vi "10-Tap 8-bit Camera with DRAM (Host).vi"() -> ()   [LabVIEW 2013]
doc: "This is the host VI for the 10-Tap 8-Bit Camera with DRAM example. This example demonstrates how to acquire images from a 10-tap, 8-bit, extended configuration, Camera Link camera and display the images on the host. This example supports area scan and line scan cameras for both continuous and finite acquisitions.\n\nThis example also demonstrates the use of DRAM as a frame buffer for very high speed acquisitions. Data packing and flow-control are also employed to maximize use of the available DRAM and FIFOs in terms of both memory space and performance.\n\nAdditionally, the example demonstrates the serial server, which allows third-party camera configuration utilities to communicate with the camera using the Camera Link serial interface while this VI is running."
uses:
  <vilib>/rvi/interface/nirviOpenFPGA/nirviOpenFPGA.xnode
  <vilib>/rvi/interface/nirviMethod/nirviMethod.xnode
  <vilib>/rvi/interface/nirviCloseFPGA/nirviCloseFPGA.xnode
  <vilib>/rvi/interface/nirviReadWriteControl/nirviReadWriteControl.xnode
  <vilib>/rvi/interface/Simulation/niFpgaSimulationCallBeginRW.vi
  <vilib>/rvi/errors/niLvFpgaAdjustHostInterfaceError.vi
  <vilib>/rvi/errors/niLvFpgaMergeErrorWithErrorCode.vi
  <vilib>/FPGAPlugInAG/Dynamic/niLvFpga_Reset_Dynamic.vi
  <vilib>/FPGAPlugInAG/Dynamic/niLvFpga_Run_Dynamic.vi
  <vilib>/FPGAPlugInAG/Dynamic/niLvFpga_ConfigureFifo_Dynamic.vi
  <vilib>/FPGAPlugInAG/Dynamic/niLvFpga_StartFifo_Dynamic.vi
  <vilib>/FPGAPlugInAG/Dynamic/niLvFpga_ReadFifo_Dynamic.vi
  <vilib>/FPGAPlugInAG/Dynamic/niLvFpga_WriteFifo_Dynamic.vi
  <vilib>/FPGAPlugInAG/Dynamic/niLvFpga_StopFifo_Dynamic.vi
  FPGA Bitfiles/10-Tap8-bitwithout_DRAM.lvbitx
  10-Tap 8-bit Camera with DRAM v2 (FPGA).vi
  <vilib>/FPGAPlugInAG/Dynamic/niLvFpga_Close_Dynamic.vi
  <vilib>/userdefined/High Color/nirio_resource_hc.ctl
panel:
  out "Data 2":u64[](array[numeric])
  out "output array 2":u8[][](array[numeric])
  out "Elements Remaining":u32
  out "Data":u64[](array[numeric])
  out "10Pixel values":T1(array[cluster])
  out "output array":u8[](array[numeric])
  out "Y Resolution":i32
  out "X Resolution":i32
  in  "Test Image Path":path=path "C:/Users/achiu/Desktop/testflyimage1.jpg"
  in  "Sim?":bool=TRUE
  in  "DMA Buffer Size\n(In Images)":u32=64 caption="DMA Buffer Size"
  in  "Signal Mapping":T2(ring)=enum."Basler 10-tap"
  out "Acq In Progress":bool
  in  "Line Scan":bool
  in  "Frames To Acquire":u32=1 caption="Frames To Acquire\n(0 = infinite)"
  in  "Cancel":bool
  out "Acq'd Frame Width":u32
  in  "Stopped":bool
  in  "RIO Device":T3="RIO1"
  out "DMA Write Timeout":bool
  in  "Start Serial Server":bool
  out "Frames Acq'd":u32
  out "Acq'd Frame Height":u32
  out "Image":T4(plugin-control)
  in  "Acquire":bool
  in  "Stop":bool
  in  "Image Height":u32=100 max=65535
  in  "Image Width":u32=120 max=65535 step=40
  out "Initialized":bool
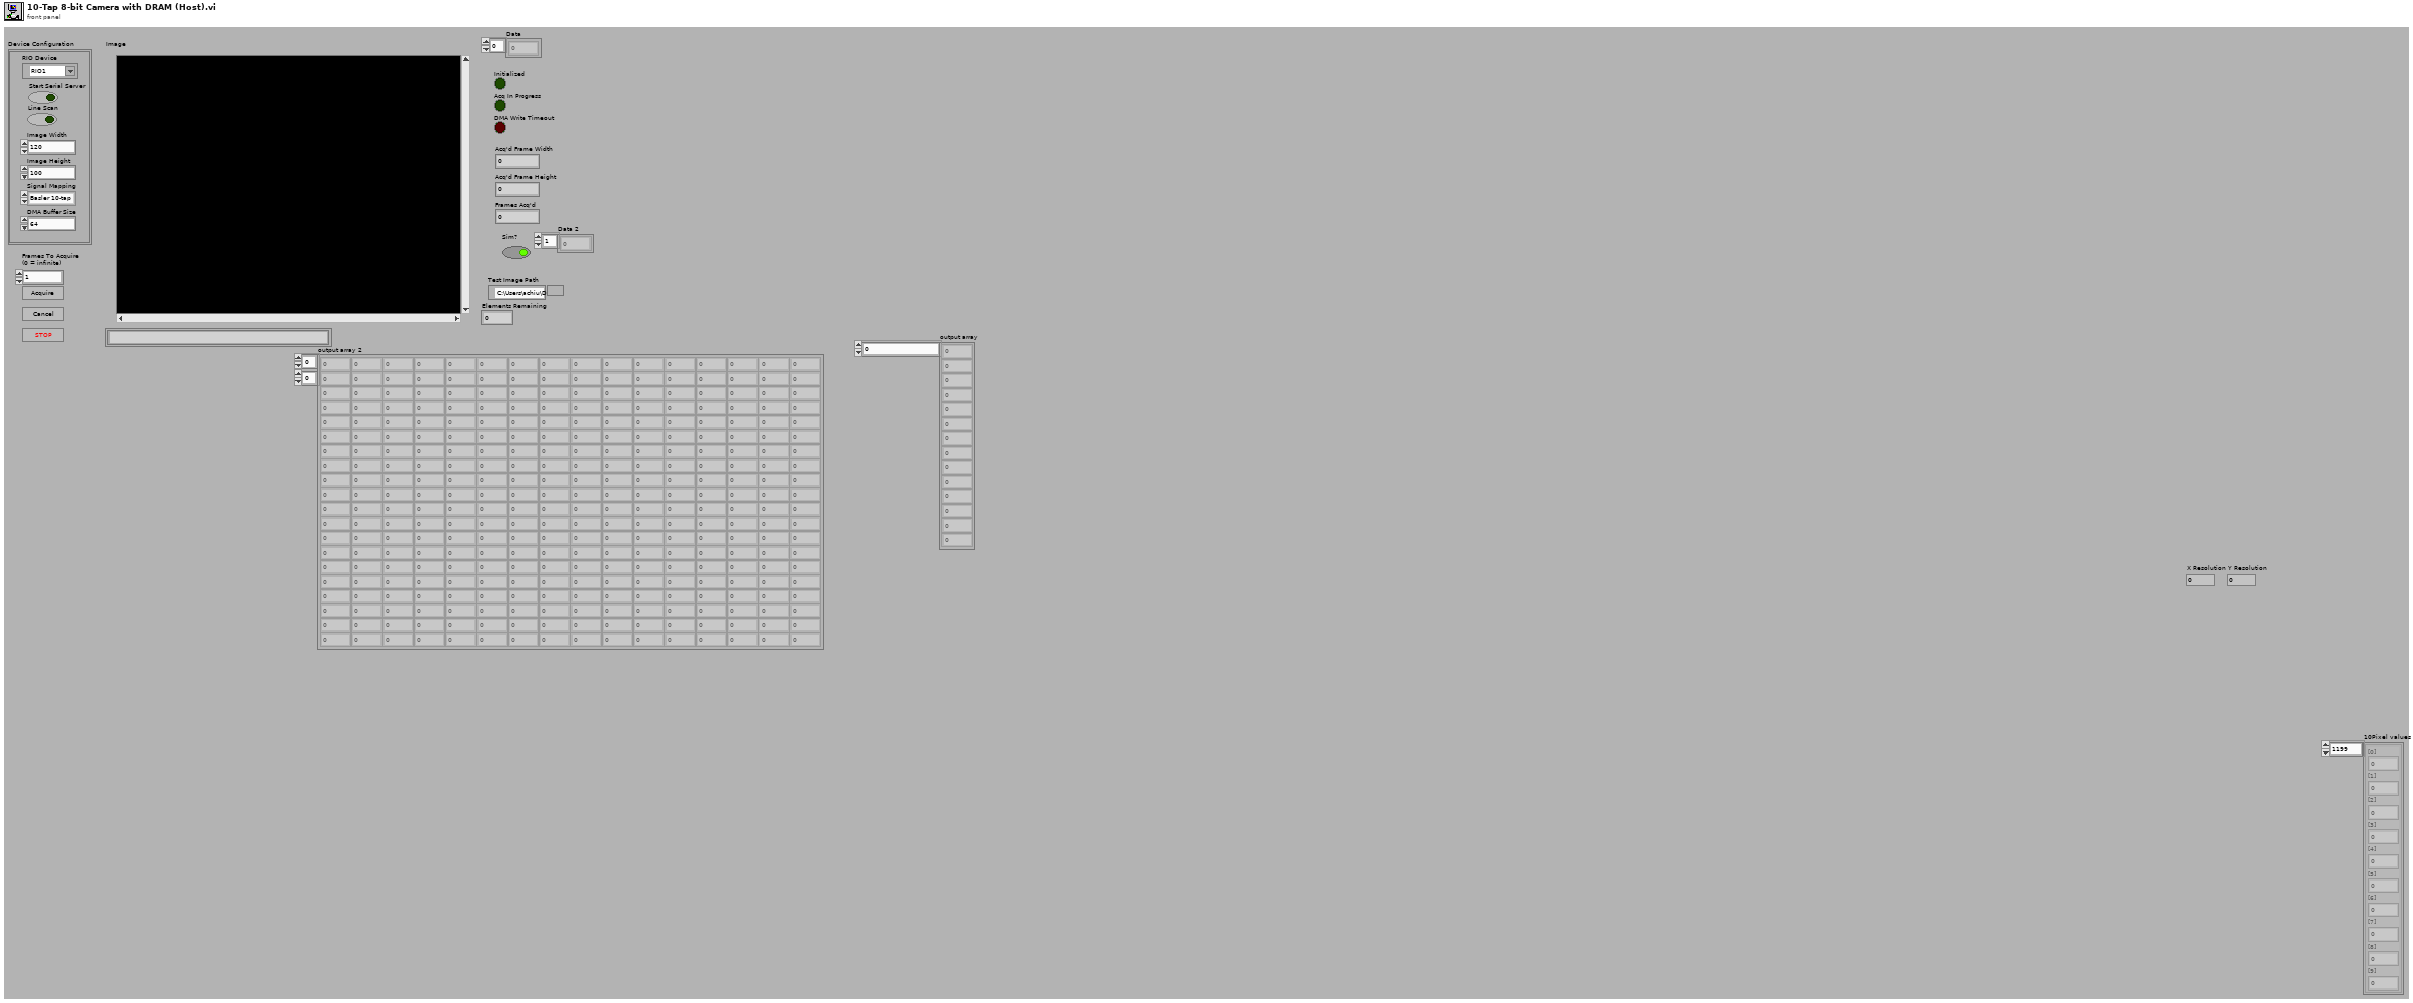
[diagram p1: front panel]
types:
  T1 = cluster{"[0]":u8, "[1]":u8, "[2]":u8, "[3]":u8, "[4]":u8, "[5]":u8, "[6]":u8, "[7]":u8, "[8]":u8, "[9]":u8}[]
  T2 = enum8{"Standard", "Basler 10-tap", "Vosskühler 10-tap"}
  T3 = typedef "nirio_resource_hc.ctl" = tag
  T4 = typedef "IMAQ Image.ctl" = refnum<image>
  T5 = typedef "Image Type" = u32
  T6 = cluster{"[0]":u8, "[1]":u8, "[2]":u8, "[3]":u8, "[4]":u8, "[5]":u8, "[6]":u8, "[7]":u8, "[8]":u8, "[9]":u8}
  T7 = enum16{"big-endian, network order", "native, host order", "little-endian"}
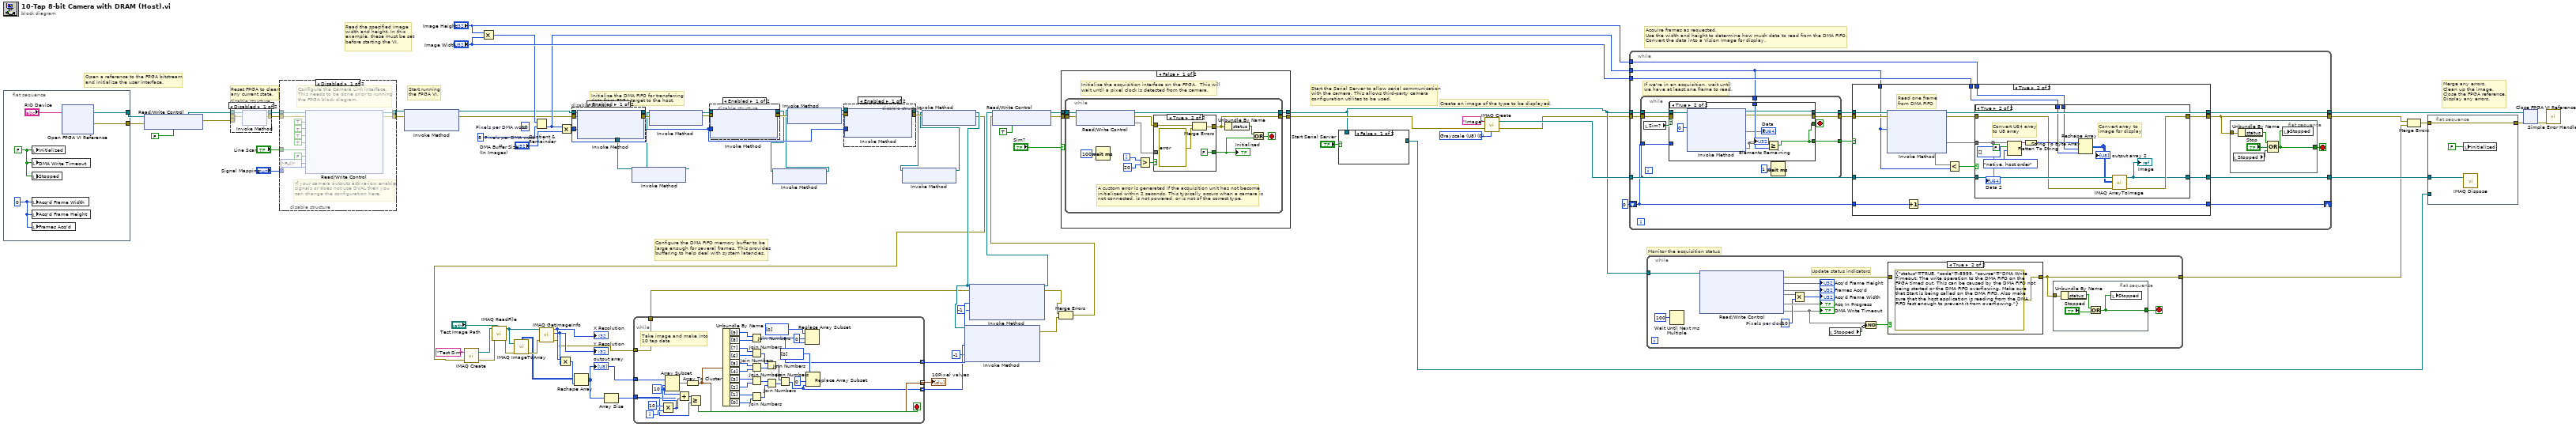
[diagram p0: block diagram]
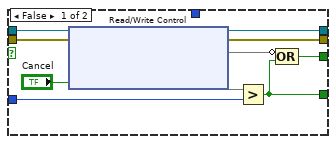
[diagram p3: hidden frame]
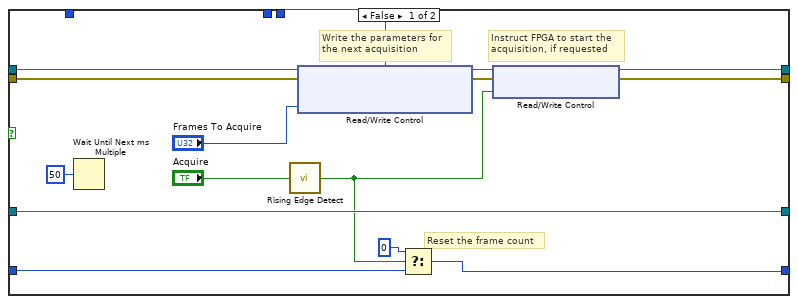
[diagram p4: hidden frame]
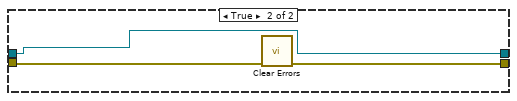
[diagram p12: hidden frame]
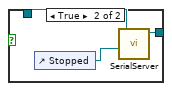
[diagram p13: hidden frame]
diagram:
  w19 = u32 8  # Pixels per DMA word
  (unwired) u32 10  # Pixels per DMA word
  w76 = T5 0 items=["Grayscale (U8)", "Grayscale (I16)", "Grayscale (SGL)", "Complex (CSG)", "RGB (U32)", "HSL (U32)", "RGB (U64)", "Grayscale (U16)"] ("Image Type")
  # "Acquire frames as requested.\nUse the width and height to determine how much data to read from the DMA FIFO.\nConvert the data into a Vision Image for display."
  # "Monitor the acquisition status"
  # "Initialize the DMA FIFO for transferring\ndata from FPGA target to the host."
  # "Configure the DMA FIFO memory buffer to be\nlarge enough for several frames. This provides\nbuffering to help deal with system latencies."
  # "Start running\nthe FPGA VI."
  # "Reset FPGA to clear\nany current state."
  # "Read the specified image\nwidth and height. In this\nexample, these must be set\nbefore starting the VI."
  # "Merge any errors.\nClean up the image.\nClose the FPGA reference.\nDisplay any errors."
  # "Start the Serial Server to allow serial communication\nwith the camera. This allows third-party camera\nconfiguration utilites to be used."
  # "Create an image of the type to be displayed."
  # "Open a reference to the FPGA bitstream\nand initialize the user interface."
  n1 = flat-sequence {
    tunnel: [w81] -> w6
    tunnel: [w80] -> w7
    frame #0 {
      w84 = u32 0 ("Num Lines Acq'd")
      w83 = FALSE ("stop")
      n2 = local write "Initialized"(w83) -> ()
      n3 = local write "DMA Write Timeout"(w83) -> ()
      n4 = local write "Stopped"(w83) -> ()
      n5 = local write "Acq'd Frame Width"(w84) -> ()
      n6 = local write "Acq'd Frame Height"(w84) -> ()
      n7 = local write "Frames Acq'd"(w84) -> ()
      n8 = xnode "Open FPGA VI Reference"("resource name"="RIO Device") -> ("FPGA VI Reference Out"=w81:refnum<k20>, "error out"=w80:errorcluster)  [unwired: 1 in]
    }
  }
  n9 = xnode "Read/Write Control"("FPGA VI Reference In"=w6, "error in"=w7, "Acq Control.Initialize"=FALSE ("Arm Acquisition")) -> ("FPGA VI Reference Out"=w5:refnum<k20>, "error out"=w4:errorcluster)
  n10 = disable-structure shown="Disabled" {
    disable-tunnel: [w85 _] -> _
    disable-tunnel: w5 -> [w88 w89]
    disable-tunnel: [w87 _] -> w64
    disable-tunnel: [w86 w89] -> w63
    disable-tunnel: w4 -> [w85 _]
    frame Disabled {
      n11 = xnode "Invoke Method"("FPGA VI Reference In"=w88, "error in"=w85) -> ("FPGA VI Reference Out"=w86:refnum<k20>, "error out"=w87:errorcluster)
    }
    frame Enabled {
    }
  }
  n12 = disable-structure shown="Disabled" {
    disable-tunnel: [w101 w103] -> w31
    disable-tunnel: w64 -> [w100 w102]
    disable-tunnel: [w99 w102] -> w30
    disable-tunnel: w63 -> [w98 w103]
    disable-tunnel: "Line Scan" -> [w93 _]
    disable-tunnel: "Signal Mapping" -> [w90 _]
    frame Disabled {
      # "If your camera outputs active-low enable\nsignals or does not use DVAL then you \ncan change the configuration here."
      # "Configure the Camera Link interface.\nThis needs to be done prior to running\nthe FPGA block diagram."
      n13 = xnode "Read/Write Control"("FPGA VI Reference In"=w98, "error in"=w100, "CL Config.FVAL Active High"=TRUE ("IO Module Config.CL FVAL Active High"), "CL Config.LVAL Active High"=TRUE ("IO Module Config.CL LVAL Active High"), "CL Config.DVAL Active High"=TRUE ("IO Module Config.CL DVAL Active High"), "CL Config.Spare Active High"=TRUE ("IO Module Config.CL Spare Active High"), "CL Config.Line Scan"=w93, "Acq Control.Ignore DVAL"=FALSE ("CL Config.Line Scan"), "CL Config.Configuration"=enum8{"Base", "Medium", "Full"}."Full", "CL Config.Signal Mapping"=w90) -> ("FPGA VI Reference Out"=w101:refnum<k20>, "error out"=w99:errorcluster)
    }
    frame Enabled {
    }
  }
  n14 = xnode "Invoke Method"("FPGA VI Reference In"=w31, "error in"=w30) -> ("FPGA VI Reference Out"=w29:refnum<k20>, "error out"=w28:errorcluster)  [unwired: 1 in]
  n15 = Multiply(x="Image Height", y="Image Width") -> (x*y=w57:u32)
  n16 = Quotient & Remainder(x=w57, y=w19) -> (floor(x/y)=w56:u32)  [unwired: 1 out]
  n17 = Multiply(x=w56, y="DMA Buffer Size\n(In Images)") -> (x*y=w55:u32)
  n18 = disable-structure shown="Enabled" {
    disable-tunnel: w29 -> [w108 w110]
    disable-tunnel: w28 -> [w107 w109]
    disable-tunnel: w55 -> [w106 _]
    disable-tunnel: [w104 w110] -> _
    disable-tunnel: [w105 w109] -> w39
    disable-tunnel: [w104 _] -> w25
    frame Enabled {
      n19 = xnode "Invoke Method"("FPGA VI Reference In"=w108, "error in"=w107, "Requested Depth"=w106) -> ("FPGA VI Reference Out"=w104:refnum<k20>, "error out"=w105:errorcluster)  [unwired: 1 out]
    }
    frame Disabled {
    }
  }
  n20 = xnode "Invoke Method"("FPGA VI Reference In"=w25) -> ("FPGA VI Reference Out"=w24:refnum<k20>)  [unwired: 1 in, 1 out]
  n21 = xnode "Invoke Method"("FPGA VI Reference In"=w24, "error in"=w39) -> ("FPGA VI Reference Out"=w37:refnum<k20>, "error out"=w35:errorcluster)
  n22 = disable-structure shown="Enabled" {
    disable-tunnel: w55 -> [w115 _]
    disable-tunnel: w37 -> [w114 w117]
    disable-tunnel: [w113 w117] -> w23
    disable-tunnel: [w112 w116] -> w36
    disable-tunnel: w35 -> [w111 w116]
    frame Enabled {
      n23 = xnode "Invoke Method"("FPGA VI Reference In"=w114, "error in"=w111, "Requested Depth"=w115) -> ("FPGA VI Reference Out"=w113:refnum<k20>, "error out"=w112:errorcluster)  [unwired: 1 out]
    }
    frame Disabled {
    }
  }
  n24 = xnode "Invoke Method"("FPGA VI Reference In"=w23) -> ("FPGA VI Reference Out"=w22:refnum<k20>)  [unwired: 1 in, 1 out]
  n25 = xnode "Invoke Method"("FPGA VI Reference In"=w22, "error in"=w36) -> ("FPGA VI Reference Out"=w34:refnum<k20>, "error out"=w33:errorcluster)
  n26 = disable-structure shown="Enabled" {
    disable-tunnel: w55 -> [w122 _]
    disable-tunnel: w34 -> [w121 w124]
    disable-tunnel: w33 -> [w120 w123]
    disable-tunnel: [w119 w124] -> w21
    disable-tunnel: [w118 w123] -> w32
    frame Enabled {
      n27 = xnode "Invoke Method"("FPGA VI Reference In"=w121, "error in"=w120, "Requested Depth"=w122) -> ("FPGA VI Reference Out"=w119:refnum<k20>, "error out"=w118:errorcluster)  [unwired: 1 out]
    }
    frame Disabled {
    }
  }
  n28 = xnode "Invoke Method"("FPGA VI Reference In"=w21) -> ("FPGA VI Reference Out"=w20:refnum<k20>)  [unwired: 1 in, 1 out]
  n29 = xnode "Invoke Method"("FPGA VI Reference In"=w20, "error in"=w32) -> ("FPGA VI Reference Out"=w14:refnum<k20>, "error out"=w13:errorcluster)
  n30 = call "IMAQ Create"("Image Name"="Test Sim", "error in (no error)"=w13) -> ("New Image"=w51:T4, "error out"=w50:errorcluster)  [unwired: 3 in]
  n31 = call "IMAQ ReadFile"("File Path"="Test Image Path", "error in (no error)"=w50, "Image"=w51) -> ("error out"=w45:errorcluster, "Image Out"=w49:T4)  [unwired: 4 in, 3 out]
  n32 = call "IMAQ ImageToArray"("error in (no error)"=w45, "Image"=w49) -> ("error out"=w44:errorcluster, "Image Pixels (U8)"=w1:u8[][])  [unwired: 2 in, 3 out]
  n33 = call "IMAQ GetImageInfo"("error in (no error)"=w44, "Image"=w49) -> ("error out"=w40:errorcluster, "Y Resolution"=w42:i32, "X Resolution"=w43:i32)  [unwired: 2 in, 5 out]
  "X Resolution" <- w43
  "Y Resolution" <- w42
  n34 = Multiply(x=w43, y=w42) -> (x*y=w41:i32)
  n35 = Reshape Array(w1, w41) -> (w47:u8[])
  "output array" <- w47
  n36 = Array Size(array=w47) -> (size(s)=w48:i32)
  n37 = while {
    tunnel: w48 -> [w150]
    tunnel: w47 -> [w155]
    tunnel: [w132] -> w46 mode=indexing
    tunnel: w40 -> [w125]
    tunnel: [w127] -> w27 mode=indexing
    tunnel: [w126] -> w26 mode=indexing
    tunnel: [w125] -> w8
    i -> [w157]
    stop <- w149 stop-if-true
    w152 = 10 ("length")
    # "Take image and make into\n10 tap data"
    n38 = Multiply(x=10, y=w157) -> (x*y=w153:i32)
    n39 = Array Subset(array=w155, index=w153, length=w152) -> (w154:u8[])
    n40 = Add(x=w152, y=w153) -> (x+y=w151:i32)
    n41 = Array To Cluster(array=w154) -> (cluster=w132:T6)
    n42 = Greater Or Equal?(x=w151, y=w150) -> (x >= y?=w149:bool)
    n43 = Unbundle By Name(w132) -> ("[9]"=w148:u8, "[8]"=w147:u8, "[7]"=w146:u8, "[6]"=w145:u8, "[5]"=w144:u8, "[4]"=w143:u8, "[3]"=w142:u8, "[2]"=w141:u8, "[1]"=w140:u8, "[0]"=w139:u8)
    n44 = Join Numbers(hi=w148, lo=w147) -> ((hi.lo)=w127:u16)
    n45 = Join Numbers(hi=w146, lo=w145) -> ((hi.lo)=w137:u16)
    n46 = Join Numbers(hi=w144, lo=w143) -> ((hi.lo)=w136:u16)
    n47 = Join Numbers(hi=w142, lo=w141) -> ((hi.lo)=w135:u16)
    n48 = Join Numbers(hi=w140, lo=w139) -> ((hi.lo)=w138:u16)
    n49 = Join Numbers(hi=w137, lo=w136) -> ((hi.lo)=w134:u32)
    n50 = Join Numbers(hi=w135, lo=w138) -> ((hi.lo)=w133:u32)
    n51 = Join Numbers(hi=w134, lo=w133) -> ((hi.lo)=w126:u64)
    n52 = Replace Array Subset(array=u16[] [0] ("Data"), new element=w127, index=0) -> ()  [unwired: 1 out]
    n53 = Replace Array Subset(array=u64[] [0] ("Data"), new element=w126, index=0) -> ()  [unwired: 1 out]
  }
  "10Pixel values" <- w46
  n54 = xnode "Invoke Method"("FPGA VI Reference In"=w14, "Data"=w26, "Timeout (ms)"=-1) -> ("error out"=w11:errorcluster)  [unwired: 1 in, 2 out]
  n55 = xnode "Invoke Method"("FPGA VI Reference In"=w14, "error in"=w8, "Data"=w27, "Timeout (ms)"=-1) -> ("FPGA VI Reference Out"=w9:refnum<k20>, "error out"=w12:errorcluster)  [unwired: 1 out]
  n56 = Merge Errors(w12, w11) -> (w10:errorcluster)
  n57 = xnode "Read/Write Control"("FPGA VI Reference In"=w9, "error in"=w10, "Acq Control.Initialize"=TRUE ("Arm Acquisition")) -> ("FPGA VI Reference Out"=w79:refnum<k20>, "error out"=w78:errorcluster)
  n58 = case shown="False" "Sim?" {
    tunnel: w79 -> [w161 w181]
    tunnel: w78 -> [w160 w182]
    tunnel: [w159 w181] -> w18
    tunnel: [w158 w183] -> w61
    frame False {
      # "Initialize the acquisition interface on the FPGA.  This will\nwait until a pixel clock is detected from the camera."
      n59 = while {
        tunnel: w161 -> [w169]
        tunnel: w160 -> [w168]
        tunnel: [w167] -> w159
        tunnel: [w171] -> w158
        i -> [w163]
        stop <- w174 stop-if-true
        # "A custom error is generated if the acquisition unit has not become\ninitialized within 2 seconds. This typically occurs when a camera is\nnot connected, is not powered, or is not of the correct type."
        n60 = xnode "Read/Write Control"("FPGA VI Reference In"=w169, "error in"=w168) -> ("FPGA VI Reference Out"=w167:refnum<k20>, "error out"=w166:errorcluster, "Acq Status.Initialized"=w165)
        n61 = Wait (ms)(milliseconds to wait=u32 100) -> ()  [unwired: 1 out]
        n62 = Greater?(x=w163, y=20) -> (0:w164:bool)
        n63 = case shown="True" w164 {
          tunnel: [w176 FALSE] -> w170
          tunnel: w165 -> [w176 _]
          tunnel: w166 -> [w175 w178]
          tunnel: [w175 w180] -> w171
          frame False {
          }
          frame True {
            n64 = Merge Errors(w178, errorcluster {"status"=TRUE, "code"=-8999, "source"="Acquisition Initialization: This error typically occurs when a camera is not properly connected, is not powered, or is not of the correct type."} ("error in")) -> (w180:errorcluster)
          }
        }
        "Initialized" <- w170
        n65 = Unbundle By Name(w171) -> ("status"=w173:bool)
        n66 = Or(x=w173, y=w170) -> (x .or. y?=w174:bool)
      }
    }
    frame True {
      n67 = call <vilib>:"Clear Errors.vi"("error in (no error)"=w182) -> ("error out"=w183:errorcluster)  [unwired: 6 in]
    }
  }
  n68 = case shown="False" "Start Serial Server" {
    tunnel: [_ w184] -> w68
    tunnel: w18 -> [_ w185]
    frame False {
    }
    frame True {
      n69 = control-ref of="Stopped"() -> (w186:refnum<vi>)
      n70 = call "SerialServer.vi"("Stop Refnum"=w186, "FPGA VI Reference In"=w185) -> ("FPGA VI Reference Out"=w184:refnum<k20>)  [unwired: 5 in]
    }
  }
  n71 = call "IMAQ Create"("Image Name"="Image", "Image Type"=w76, "error in (no error)"=w61) -> ("New Image"=w59:T4, "error out"=w15:errorcluster)  [unwired: 2 in]
  n72 = while {
    tunnel: w18 -> [w194]
    tunnel: w15 -> [w193]
    tunnel: w56 -> [w187]
    tunnel: "Image Height" -> [w201]
    tunnel: "Image Width" -> [w200]
    tunnel: w59 -> [w199]
    tunnel: [w197] -> w66
    tunnel: [w198] -> w75
    tunnel: [w195] -> w70
    shift-right: [w189] -> _
    shift-left: u32 0 -> [w188]
    stop <- w196 stop-if-true
    # "If we're in an acquisition, wait until\nwe have at least one frame to read."
    n73 = while {
      tunnel: w194 -> [w208]
      tunnel: w193 -> [w207]
      tunnel: [w205] -> w192
      tunnel: [w206] -> w191
      tunnel: w188 -> [w211]
      tunnel: [w209] -> w190
      tunnel: w187 -> [w203]
      stop <- w210 stop-if-true
      n74 = local read "Sim?"() -> (w204:bool)
      n75 = case shown="True" w204 {
        tunnel: w211 -> [w221 _]
        tunnel: [w220 w222] -> w210
        tunnel: [w219 w222] -> w209
        tunnel: w208 -> [w218 w229]
        tunnel: w207 -> [w217 _]
        tunnel: [w216 w225] -> w206
        tunnel: [w215 w224] -> w205
        tunnel: w203 -> [_ w226]
        frame False {
          n76 = xnode "Read/Write Control"("FPGA VI Reference In"=w218, "error in"=w217, "Acq Control.Cancel Acq"="Cancel") -> ("FPGA VI Reference Out"=w216:refnum<k20>, "error out"=w215:errorcluster, "Acq Status.Acq In Progress"=w214, "Acq Status.Frames Acq'd"=w213)
          n77 = Greater?(x=w213, y=w221) -> (0:w219:bool)
          n78 = Compound Arithmetic op=OR(invert w214, w219) -> (w220:bool)
        }
        frame True {
          n79 = xnode "Invoke Method"("FPGA VI Reference In"=w229, "Number of Elements"=u32 0) -> ("FPGA VI Reference Out"=w225:refnum<k20>, "error out"=w224:errorcluster, "Data"=→"Data":void[], "Elements Remaining"=w227)  [unwired: 2 in]
          "Elements Remaining" <- w227
          n80 = Greater Or Equal?(x=w227, y=w226) -> (x >= y?=w222:bool)
        }
      }
      n81 = Wait (ms)(milliseconds to wait=u32 1) -> ()  [unwired: 1 out]
    }
    n82 = case shown="True" w190 {
      tunnel: w191 -> [w245 w257]
      tunnel: w192 -> [w244 w256]
      tunnel: w187 -> [_ w250]
      tunnel: w201 -> [w238 w264]
      tunnel: w200 -> [_ w263]
      tunnel: w199 -> [w249 w262]
      tunnel: [w240 w260] -> w197
      tunnel: [w243 w259] -> w198
      tunnel: [w249 w258] -> w195
      tunnel: w188 -> [w246 w255]
      tunnel: [w248 w254] -> w189
      frame False {
        # "Reset the frame count"
        # "Instruct FPGA to start the\nacquisition, if requested"
        # "Write the parameters for\nthe next acquisition"
        n83 = Wait Until Next ms Multiple(millisecond multiple=u32 50) -> ()  [unwired: 1 out]
        n84 = call "Rising Edge Detect.vi"("Input"="Acquire") -> ("Pulse"=w235:bool)  [unwired: 4 in]
        n85 = xnode "Read/Write Control"("FPGA VI Reference In"=w245, "error in"=w244, "Acq Control.Line Scan Height"=w238, "Acq Control.Frames To Acq"="Frames To Acquire") -> ("FPGA VI Reference Out"=w242:refnum<k20>, "error out"=w241:errorcluster)
        n86 = Select(t=u32 0, s=w235, f=w246) -> (s? t:f=w248:u32)
        n87 = xnode "Read/Write Control"("FPGA VI Reference In"=w242, "error in"=w241, "Acq Control.Acquire"=w235) -> ("FPGA VI Reference Out"=w243:refnum<k20>, "error out"=w240:errorcluster)
      }
      frame True {
        # "Read one frame\nfrom DMA FIFO"
        n88 = xnode "Invoke Method"("FPGA VI Reference In"=w257, "error in"=w256, "Number of Elements"=w250) -> ("FPGA VI Reference Out"=w259:refnum<k20>, "error out"=w261:errorcluster, "Data"=w253:void[], "Elements Remaining"=w251)  [unwired: 1 in]
        n89 = Increment(x=w255) -> (x+1=w254:u32)
        n90 = Less?(x=w251, y=w250) -> (x < y?=w252:bool)
        n91 = case shown="True" w252 {
          tunnel: w264 -> [_ w278]
          tunnel: w263 -> [_ w277]
          tunnel: w262 -> [w266 w276]
          tunnel: w261 -> [w265 w275]
          tunnel: [w265 w274] -> w260
          tunnel: [w266 w273] -> w258
          tunnel: w253 -> [_ w270]
          frame False {
            # "Do not display the image if we're falling behind in the acquisition."
          }
          frame True {
            (unwired) u64[] [] ("Data")
            # "Convert U64 array\nto U8 array"
            # "Convert array to\nimage for display"
            n92 = Flatten To String(anything=w270, prepend array or string size? (T)=FALSE, byte order (0:big-endian, network order)=T7."native, host order") -> (data string=w268:string)  [unwired: 1 in, 2 out]
            n93 = String To Byte Array(string=w268) -> (unsigned byte array=w267:u8[])
            n94 = Reshape Array(w267, w278, w277) -> (w272:u8[][])
            "output array 2" <- w272
            n95 = call "IMAQ ArrayToImage"("error in (no error)"=w275, "Image Pixels (U8)"=w272, "Image"=w276) -> ("error out"=w274:errorcluster, "Image Out"=w273:T4)  [unwired: 7 in]
            "Image" <- w273
            "Data 2" <- w270
          }
        }
      }
    }
    n96 = flat-sequence {
      tunnel: w197 -> [w232]
      tunnel: [w231] -> w196
      frame #0 {
        n97 = local read "Stopped"() -> (w230:bool)
        n98 = Unbundle By Name(w232) -> ("status"=w233:bool)
        n99 = Compound Arithmetic op=OR(w233, "Stop", w230) -> (w231:bool)
        n100 = local write "Stopped"(w231) -> ()
      }
    }
  }
  n101 = while {
    tunnel: w18 -> [w289]
    tunnel: [w292] -> w65
    stop <- w291 stop-if-true
    w282 = u32 10  # Pixels per clock
    # "Update status indicators"
    n102 = Wait Until Next ms Multiple(millisecond multiple=u32 100) -> ()  [unwired: 1 out]
    n103 = xnode "Read/Write Control"("FPGA VI Reference In"=w289) -> ("error out"=w288:errorcluster, "Acq Status.Lines Per Frame"=→"Acq'd Frame Height", "Acq Status.Frames Acq'd"=→"Frames Acq'd", "Acq Status.Clocks Per Line"=w283, "Acq Status.Acq In Progress"=→"Acq In Progress", "Acq Status.DMA Write Timeout"=w280)  [unwired: 1 in, 1 out]
    "DMA Write Timeout" <- w280
    n104 = Multiply(x=w283, y=w282) -> (x*y=→"Acq'd Frame Width":u32)
    n105 = local read "Stopped"() -> (w279:bool)
    n106 = Compound Arithmetic op=AND(w280, invert w279) -> (w281:bool)
    n107 = case shown="True" w281 {
      tunnel: w288 -> [w297 _]
      tunnel: [w297 errorcluster {"status"=TRUE, "code"=-8999, "source"="DMA Write Timeout: The write operation to the DMA FIFO on the FPGA timed out. This can be caused by the DMA FIFO not being started or the DMA FIFO overflowing. Make sure that Start is being called on the DMA FIFO. Also make sure that the host application is reading from the DMA FIFO fast enough to prevent it from overflowing."} ("error out")] -> w292
      frame False {
      }
      frame True {
      }
    }
    n108 = flat-sequence {
      tunnel: w292 -> [w296]
      tunnel: [w294] -> w291
      frame #0 {
        n109 = Unbundle By Name(w296) -> ("status"=w295:bool)
        n110 = Or(x=w295, y="Stopped") -> (x .or. y?=w294:bool)
        n111 = local write "Stopped"(w294) -> ()
      }
    }
  }
  n112 = Merge Errors(w66, w65) -> (w67:errorcluster)
  n113 = flat-sequence {
    tunnel: w67 -> [w300]
    tunnel: [w300] -> w72
    tunnel: w70 -> [w301]
    tunnel: w68 -> [_]
    frame #0 {
      n114 = local write "Initialized"(FALSE ("Module Enabled")) -> ()
      n115 = call "IMAQ Dispose"("Image"=w301) -> ()  [unwired: 5 in, 1 out]
    }
  }
  n116 = xnode "Close FPGA VI Reference"("FPGA VI Reference In"=w75, "error in"=w72) -> ("error out"=w69:errorcluster)
  n117 = call <vilib>:"Simple Error Handler.vi"("error in (no error)"=w69) -> ()  [unwired: 4 in, 5 out]
